vi "InitializeDevice.vi"(8 "error in (no error)":errorcluster, 11 "HP3458aDMM in":refnum<class "HP3458aDMM.lvclass">) -> (0 "error out":errorcluster, 3 "HP3458aDMM out":refnum<class "HP3458aDMM.lvclass">)   [LabVIEW 2014, in "SamplerPlugins.lvlib" / "HP3458aDMM.lvclass"]
uses:
  HP3458aDMM.lvclass
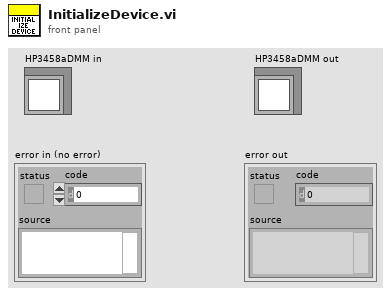
[diagram p1: front panel]
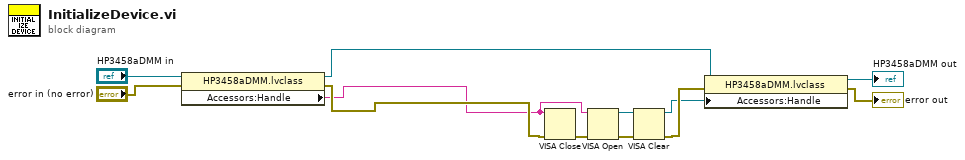
[diagram p0: block diagram]
diagram:
  n1 = property class="HP3458aDMM.lvclass"(reference="HP3458aDMM in", error in="error in (no error)") -> (reference out=w9:refnum<class "HP3458aDMM.lvclass">, error out=w2:errorcluster, "Accessors:Handle"=w1:string)
  n2 = VISA Close(VISA resource name=w1, error in (no error)=w2) -> (error out=w3:errorcluster)
  n3 = VISA Open(error in (no error)=w3, VISA resource name=w1) -> (VISA resource name=w7:refnum<visa-resource-name>, error out=w6:errorcluster)  [unwired: 3 in]
  n4 = VISA Clear(VISA resource name=w7, error in (no error)=w6) -> (VISA resource name out=w4:refnum<visa-resource-name>, error out=w5:errorcluster)
  n5 = property class="HP3458aDMM.lvclass"(reference=w9, error in=w5, "Accessors:Handle"=w4) -> (reference out=→"HP3458aDMM out":refnum<class "HP3458aDMM.lvclass">, error out=→"error out":errorcluster)
